vi "Apply General Configuration.vi"(7 "Restart (T)":bool=TRUE, 8 "error in (no error)":errorcluster, 9 "Cell Inhibit Enable":bool, 10 "Protocol (Legacy)":T1, 11 "Ethernet in":refnum<class "ENET_BS1200.lvclass">) -> (0 "error out":errorcluster, 3 "Ethernet out":refnum<class "ENET_BS1200.lvclass">)   [LabVIEW 2021, in "BS120x Driver.lvlib" / "ENET_BS1200.lvclass"]
doc: "Sends the configuration updates to the Battery Simulator 1200. Changes will not be applied until after the unit is restarted. To apply multilple configuration settings in one set, set <b>Restart</b> to false on all Settings VIs except the last one.\n(c) 2019 Bloomy Controls, Inc. All rights reserved."
uses:
  ENET_BS1200.lvclass
  TypeDefs/Protocol.ctl
  ENET_BS1200.lvclass/ENET_BS1200.ctl
  <vilib>/WebDAVClient/Advanced/Get Buffer.vi
  <vilib>/WebDAVClient/Advanced/Put Buffer.vi
  <vilib>/WebDAVClient/NI_WebDAV.lvlib
  BS120x.lvclass
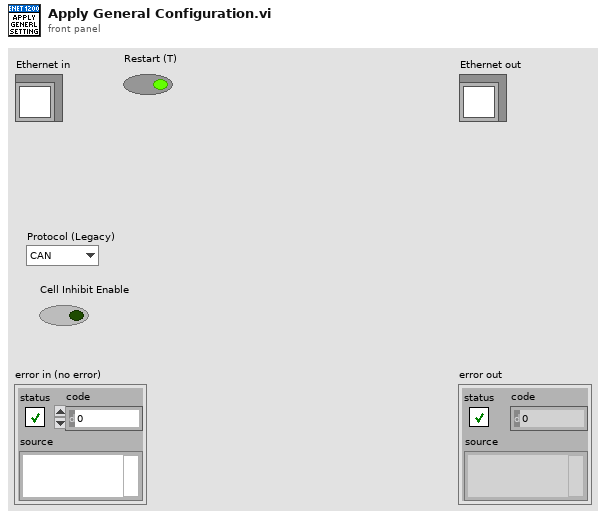
[diagram p1: front panel]
types:
  T1 = typedef "BS120x Driver.lvlib/BS120x.lvclass/Protocol.ctl" = enum16{"CAN", "Ethernet"}
  T2 = typedef "NI_WebDAV.lvlib/SessionHandle.ctl" = refnum<k1>
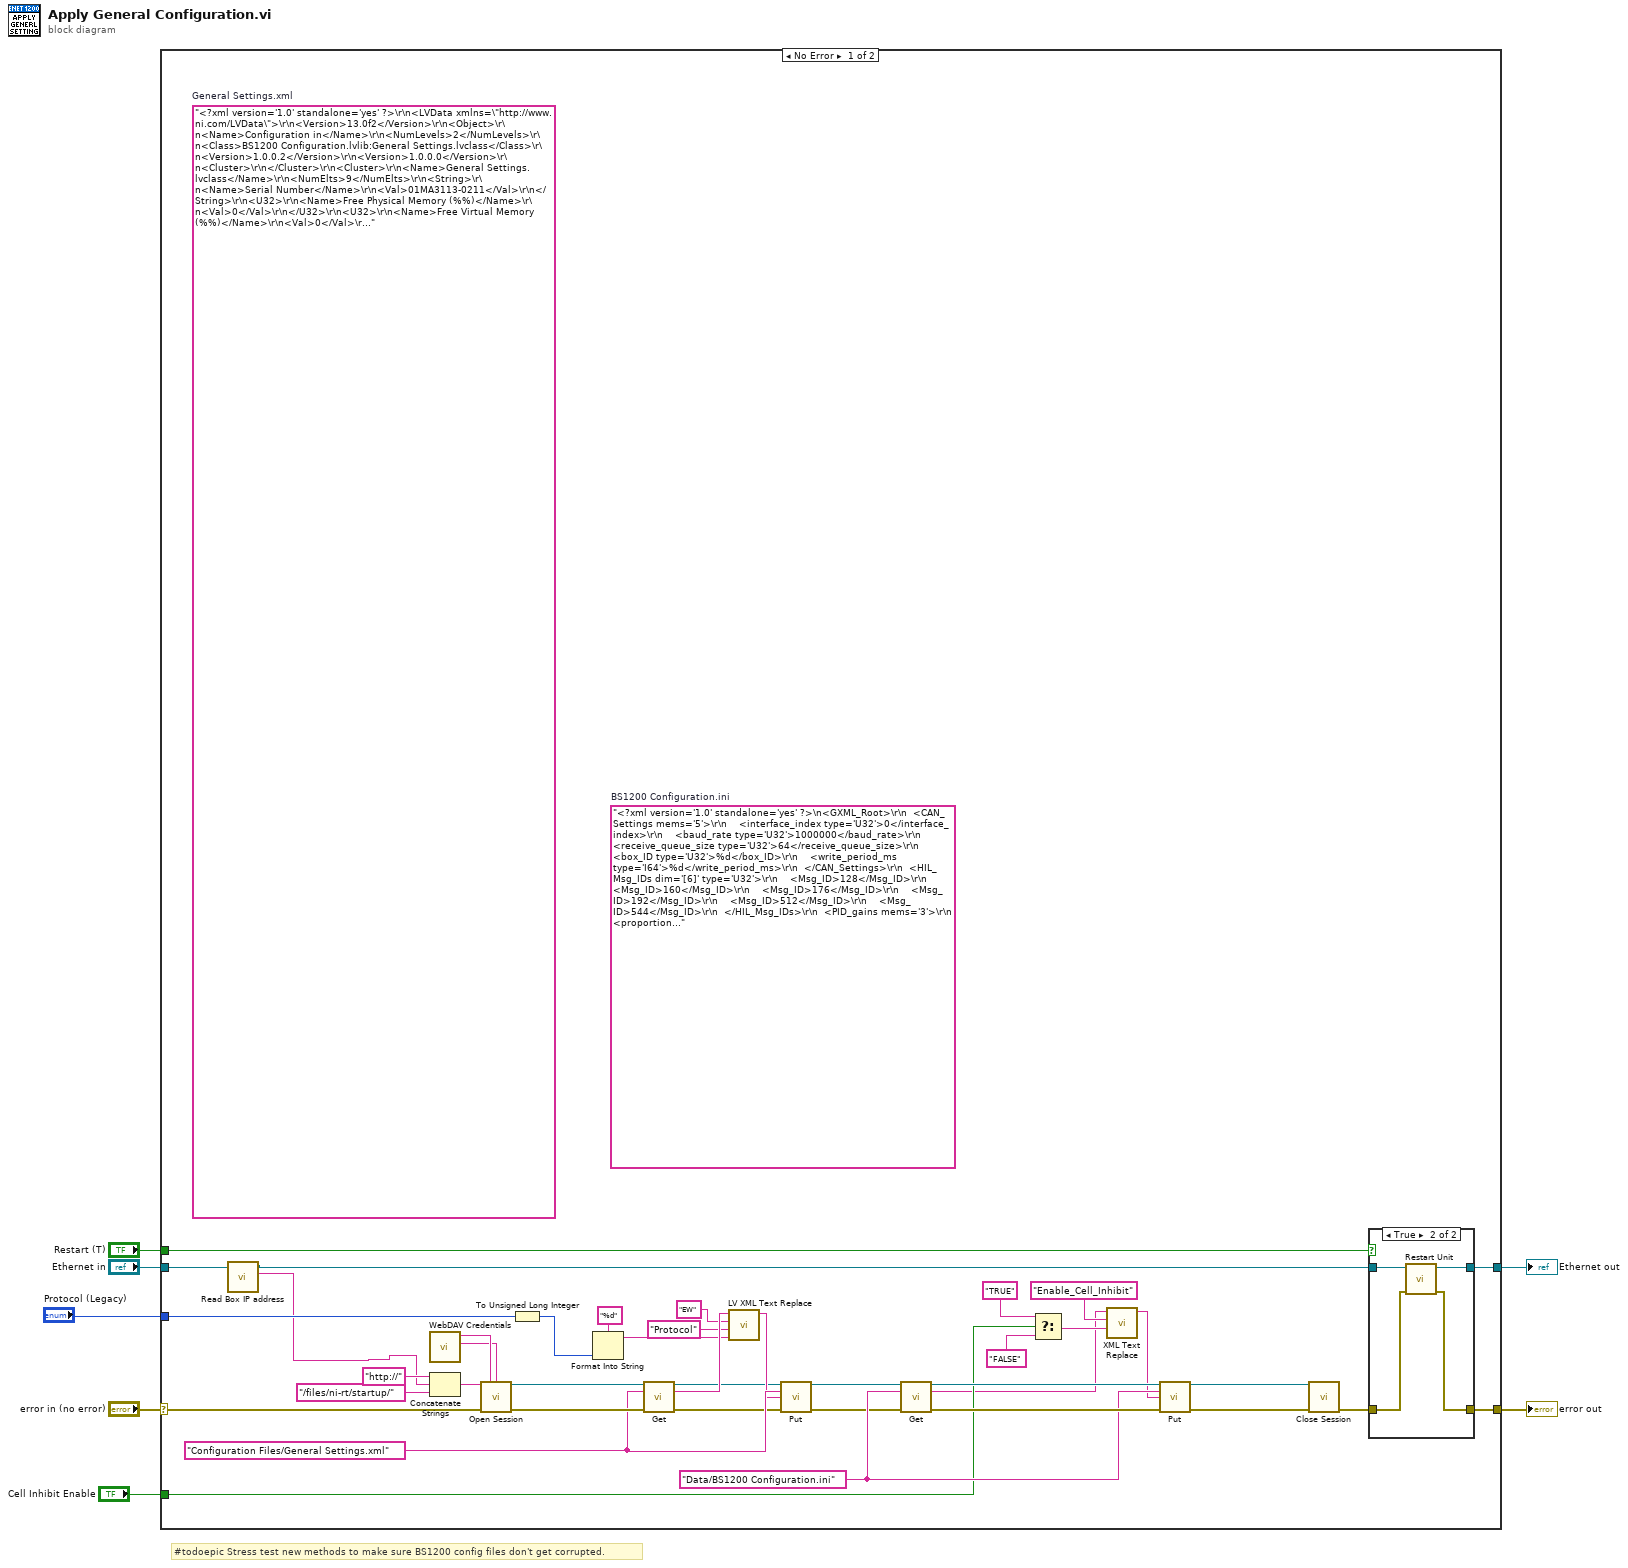
[diagram p0: block diagram]
diagram:
  # "#todoepic Stress test new methods to make sure BS1200 config files don't get corrupted."
  n1 = case shown="No Error" "error in (no error)" {
    selector: "error in (no error)" -> [w45 w55]
    tunnel: [w39 w55] -> w6
    tunnel: [w40 w54] -> w4
    tunnel: "Ethernet in" -> [w24 w54]
    tunnel: "Restart (T)" -> [w38 _]
    tunnel: "Protocol (Legacy)" -> [w25 _]
    tunnel: "Cell Inhibit Enable" -> [w12 _]
    frame No Error {
      w20 = "Data/BS1200 Configuration.ini" ("string")
      (unwired) "<?xml version='1.0' standalone='yes' ?>\n<GXML_Root>\r\n  <CAN_Settings mems='5'>\r\n    <interface_index type='U32'>0</interface_index>\r\n    <baud_rate type='U32'>1000000</baud_rate>\r\n    <receive_queue_size type='U32'>64</receive_queue_size>\r\n    <box_ID type='U32'>%d</box_ID>\r\n    <write_period_ms type='I64'>%d</write_period_ms>\r\n  </CAN_Settings>\r\n  <HIL_Msg_IDs dim='[6]' type='U32'>\r\n    <Msg_ID>128</Msg_ID>\r\n    <Msg_ID>160</Msg_ID>\r\n    <Msg_ID>176</Msg_ID>\r\n    <Msg_ID>192</Msg_ID>\r\n    <Msg_ID>512</Msg_ID>\r\n    <Msg_ID>544</Msg_ID>\r\n  </HIL_Msg_IDs>\r\n  <PID_gains mems='3'>\r\n    <proportional_gain type='DBL'>0.3</proportional_gain>\r\n    <integral_gain type='DBL'>0.55</integral_gain>\r\n    <derivative_gain type='DBL'>0</derivative_gain>\r\n  </PID_gains>\r\n  <Enable_Cell_Inhibit type='Bool'>FALSE</Enable_Cell_Inhibit>\r\n</GXML_Root>"  # BS1200 Configuration.ini
      (unwired) "<?xml version='1.0' standalone='yes' ?>\r\n<LVData xmlns=\"http://www.ni.com/LVData\">\r\n<Version>13.0f2</Version>\r\n<Object>\r\n<Name>Configuration in</Name>\r\n<NumLevels>2</NumLevels>\r\n<Class>BS1200 Configuration.lvlib:General Settings.lvclass</Class>\r\n<Version>1.0.0.2</Version>\r\n<Version>1.0.0.0</Version>\r\n<Cluster>\r\n</Cluster>\r\n<Cluster>\r\n<Name>General Settings.lvclass</Name>\r\n<NumElts>9</NumElts>\r\n<String>\r\n<Name>Serial Number</Name>\r\n<Val>01MA3113-0211</Val>\r\n</String>\r\n<U32>\r\n<Name>Free Physical Memory (%%)</Name>\r\n<Val>0</Val>\r\n</U32>\r\n<U32>\r\n<Name>Free Virtual Memory (%%)</Name>\r\n<Val>0</Val>\r\n</U32>\r\n<String>\r\n<Name>Firmware Revision</Name>\r\n<Val>1.4.0</Val>\r\n</String>\r\n<Timestamp>\r\n<Name>Calibration Date</Name>\r\n<Cluster>\r\n<Name></Name>\r\n<NumElts>4</NumElts>\r\n<I32>\r\n<Name></Name>\r\n<Val>0</Val>\r\n</I32>\r\n<I32>\r\n<Name></Name>\r\n<Val>-816713016</Val>\r\n</I32>\r\n<I32>\r\n<Name></Name>\r\n<Val>-1874952192</Val>\r\n</I32>\r\n<I32>\r\n<Name></Name>\r\n<Val>0</Val>\r\n</I32>\r\n</Cluster>\r\n</Timestamp>\r\n<EW>\r\n<Name>Protocol</Name>\r\n<Choice>CAN</Choice>\r\n<Choice>TCPIP</Choice>\r\n<Val>1</Val>\r\n</EW>\r\n<Boolean>\r\n<Name>Configured Flag</Name>\r\n<Val>1</Val>\r\n</Boolean>\r\n<Boolean>\r\n<Name>FTP Enabled</Name>\r\n<Val>0</Val>\r\n</Boolean>\r\n<Boolean>\r\n<Name>Aux IO</Name>\r\n<Val>1</Val>\r\n</Boolean>\r\n</Cluster>\r\n</Object>\r\n</LVData>"  # General Settings.xml
      w34 = "Configuration Files/General Settings.xml" ("string")
      n2 = call-dynamic "Read Box IP address.vi"("ENET_BS120x in"=w24) -> ("Box IP address"=w22:string, "ENET_BS120x out"=w23:refnum<class "ENET_BS1200.lvclass">)  [unwired: 8 in, 1 out]
      n3 = call "WebDAV Credentials.vi"() -> ("Password"=w43:string, "Username"=w44:string)  [unwired: 10 in]
      n4 = Concatenate Strings("http://" ("string"), w22, "/files/ni-rt/startup/" ("string")) -> (w42:string)
      n5 = call <vilib>:"Open Session.vi"("host uri prefix"=w42, "username"=w44, "password"=w43, "error in (no error)"=w45) -> ("session handle out"=w37:T2, "error out"=w35:errorcluster)  [unwired: 10 in]
      n6 = To Unsigned Long Integer(number=w25) -> (unsigned 32bit integer=w36:u32)
      n7 = Format Into String(format string="%d", w36) -> (resulting string=w26:string)  [unwired: 2 in, 1 out]
      n8 = call-poly <vilib>:"Get.vi"("session handle"=w37, "relative uri"=w34, "error in (no error)"=w35) -> ("session handle out"=w28:T2, "data"=w33:string, "error out"=w29:errorcluster)  [unwired: 10 in]
      n9 = call "LV XML Text Replace.vi"("Text"=w26, "Tag"="Protocol", "Datatype"="EW", "LV XML in"=w33) -> ("LV XML out"=w32:string)  [unwired: 7 in]
      n10 = call-poly <vilib>:"Put.vi"("session handle"=w28, "relative uri"=w34, "data"=w32, "error in (no error)"=w29) -> ("session handle out"=w19:T2, "error out"=w17:errorcluster)  [unwired: 10 in]
      n11 = call-poly <vilib>:"Get.vi"("session handle"=w19, "relative uri"=w20, "error in (no error)"=w17) -> ("session handle out"=w18:T2, "data"=w9:string, "error out"=w21:errorcluster)  [unwired: 10 in]
      n12 = Select(t="TRUE", s=w12, f="FALSE") -> (s? t:f=w10:string)
      n13 = call "XML Text Replace.vi"("Text"=w10, "Tag"="Enable_Cell_Inhibit", "XML in"=w9) -> ("XML out"=w13:string)  [unwired: 8 in]
      n14 = call-poly <vilib>:"Put.vi"("session handle"=w18, "relative uri"=w20, "data"=w13, "error in (no error)"=w21) -> ("session handle out"=w16:T2, "error out"=w15:errorcluster)  [unwired: 10 in]
      n15 = call <vilib>:"Close Session.vi"("session handle"=w16, "error in (no error)"=w15) -> ("error out"=w41:errorcluster)  [unwired: 13 in]
      n16 = case shown="True" w38 {
        tunnel: [w49 w50] -> w39
        tunnel: [w48 w52] -> w40
        tunnel: w41 -> [w49 w51]
        tunnel: w23 -> [w48 w53]
        frame False {
        }
        frame True {
          n17 = call-dynamic "Restart Unit.vi"("error in (no error)"=w51, "ENET in"=w53) -> ("error out"=w50:errorcluster, "ENET out"=w52:refnum<class "ENET_BS1200.lvclass">)  [unwired: 8 in]
        }
      }
    }
    frame Error {
    }
  }
  "error out" <- w6
  "Ethernet out" <- w4
